vi "setState.vi"(8 "error in (no error)":errorcluster, 10 "State":bool, 11 "Sensor in":refnum<class "Sensor.lvclass">) -> (0 "error out":errorcluster, 3 "Sensor out":refnum<class "Sensor.lvclass">)   [LabVIEW 2018, in "Sensor.lvclass"]
uses:
  Sensor.lvclass
  Sensor.lvclass/Sensor.ctl
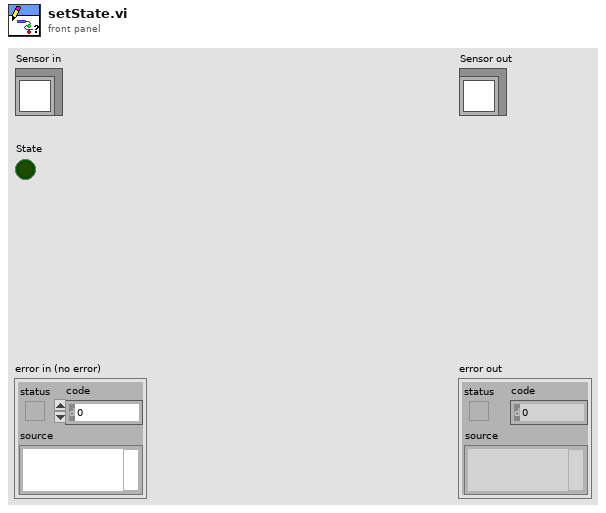
[diagram p1: front panel]
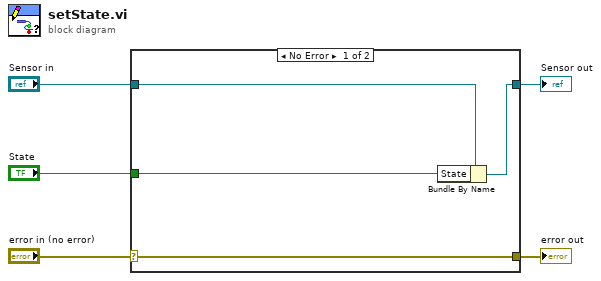
[diagram p0: block diagram]
diagram:
  n1 = case shown="No Error" "error in (no error)" {
    selector: "error in (no error)" -> [w9 w10]
    tunnel: [w9 w10] -> w4
    tunnel: [w7 w11] -> w2
    tunnel: "Sensor in" -> [w8 w11]
    tunnel: "State" -> [w6 _]
    frame No Error {
      n2 = Bundle By Name(cluster=w8, "State"=w6) -> (w7:refnum<class "Sensor.lvclass">)
    }
    frame Error {
    }
  }
  "error out" <- w4
  "Sensor out" <- w2
